vi "PH_ImageOperator.Fit Gauss.vi"(0 "No Offset?":bool, 1 "Diam":dbl, 2 "Trace":cluster{"Index":sgl[], "Trace":sgl[]}, 3 "calibrated?":bool, 4 "Order":i32, 5 "error in (no error)":errorcluster) -> (16 "Output":cluster{"Index":sgl[], "Best Fit":dbl[]}, 17 "mse":dbl format="%.2e", 18 "Best Fit Coefficients":dbl[](array[numeric]) format="%.2f", 19 "error out":errorcluster)   [LabVIEW 2014, in "PH_ImageOperator.lvlib"]
doc: "This VI fits a GAUSS function symmetrical to y-axis to the data connected to \"Trace\": a*exp(-(x/b))^2n + c\n\nwhere n is the \"Order\". To help the procedure, the \"Diameter\" (b) should be connected, while a first guess for a and c are extracted from the trace (maximum value and first value). The number of iterations is fixed to 20. The best (last) coefficients are given out as an array in the oder a, b, and c, as well as the medium square error (\"mse\")."
uses:
  PH_ImageOperator.lvlib
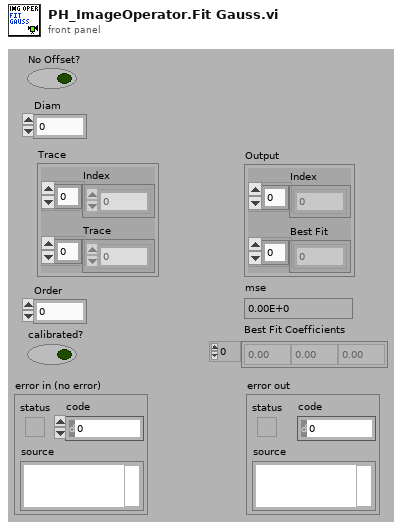
[diagram p1: front panel]
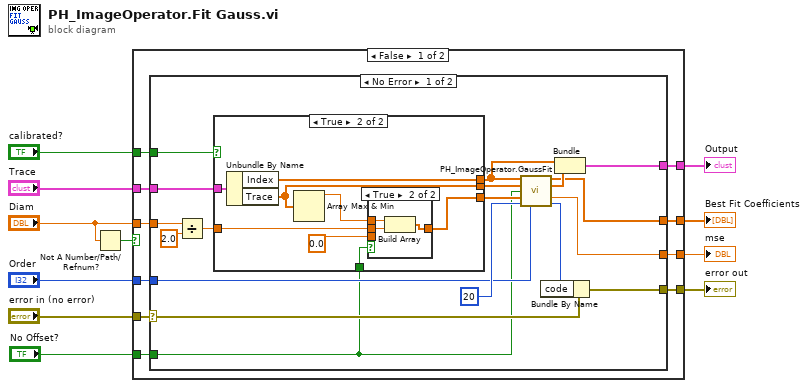
[diagram p0: block diagram]
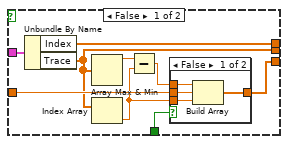
[diagram p2: hidden frame]
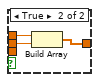
[diagram p3: hidden frame]
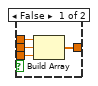
[diagram p4: hidden frame]
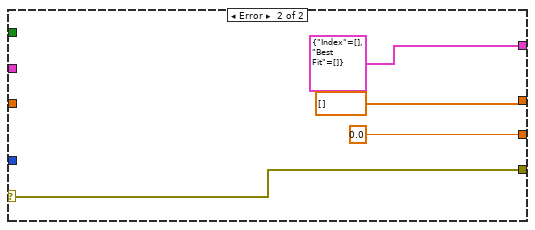
[diagram p5: hidden frame]
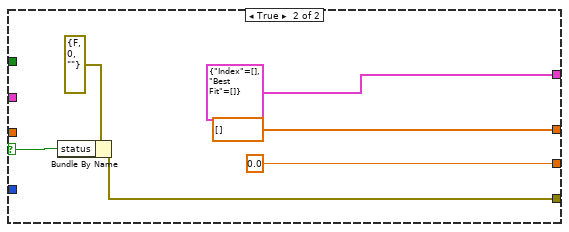
[diagram p6: hidden frame]
diagram:
  n1 = Not A Number/Path/Refnum?(number/path/refnum="Diam") -> (NaN/Path/Refnum?=w3:bool)
  n2 = case shown="False" w3 {
    selector: w3 -> [_ w78]
    tunnel: [w21 cluster{"Index":sgl[], "Best Fit":dbl[]} {"Index"=[], "Best Fit"=[]}] -> w11
    tunnel: "Trace" -> [w20 _]
    tunnel: "Order" -> [w19 _]
    tunnel: [w18 0.0 ("mse")] -> w8
    tunnel: [w17 dbl[] [] ("Best Fit Coefficients")] -> w7
    tunnel: "error in (no error)" -> [w16 _]
    tunnel: [w15 w79] -> w5
    tunnel: "Diam" -> [w14 _]
    tunnel: "calibrated?" -> [w13 _]
    tunnel: "No Offset?" -> [w12 _]
    frame False {
      n3 = case shown="No Error" w16 {
        selector: w16 -> [w28 w72]
        tunnel: w14 -> [w38 _]
        tunnel: [w34 cluster{"Index":sgl[], "Best Fit":dbl[]} {"Index"=[], "Best Fit"=[]}] -> w21
        tunnel: w20 -> [w31 _]
        tunnel: w19 -> [w23 _]
        tunnel: [w30 0.0 ("mse")] -> w18
        tunnel: [w29 dbl[] [] ("Best Fit Coefficients")] -> w17
        tunnel: [w27 w72] -> w15
        tunnel: w13 -> [w25 _]
        tunnel: w12 -> [w22 _]
        frame No Error {
          n4 = Divide(x=w38, y=2.0) -> (x/y=w37:dbl)
          n5 = case shown="True" w25 {
            tunnel: w37 -> [w48 w63]
            tunnel: [w47 w61] -> w36
            tunnel: [w46 w60] -> w35
            tunnel: [w45 w59] -> w33
            tunnel: w31 -> [w44 w58]
            tunnel: w22 -> [w40 w56]
            frame False {
              n6 = Unbundle By Name(w44) -> ("Index"=w45:sgl[], "Trace"=w47:sgl[])
              n7 = Array Max & Min(array=w47) -> (max value=w42:sgl)  [unwired: 3 out]
              n8 = Index Array(array=w47) -> (element=w43:sgl)  [unwired: 1 in]
              n9 = Subtract(x=w42, y=w43) -> (x-y=w41:sgl)
              n10 = case shown="False" w40 {
                tunnel: w48 -> [w52 w55]
                tunnel: [w51 w54] -> w46
                tunnel: w43 -> [w50 _]
                tunnel: w41 -> [w49 w53]
                frame False {
                  n11 = Build Array(w49, w52, w50) -> (w51:dbl[])
                }
                frame True {
                  n12 = Build Array(w53, w55) -> (w54:dbl[])
                }
              }
            }
            frame True {
              n13 = Unbundle By Name(w58) -> ("Index"=w59:sgl[], "Trace"=w61:sgl[])
              n14 = Array Max & Min(array=w61) -> (max value=w62:sgl)  [unwired: 3 out]
              n15 = case shown="True" w56 {
                tunnel: w63 -> [w67 w70]
                tunnel: w62 -> [w66 w69]
                tunnel: [w65 w68] -> w60
                tunnel: 0.0 ("element") -> [w64 _]
                frame False {
                  n16 = Build Array(w66, w67, w64) -> (w65:dbl[])
                }
                frame True {
                  n17 = Build Array(w69, w70) -> (w68:dbl[])
                }
              }
            }
          }
          n18 = call "PH_ImageOperator.GaussFit.vi"("Index"=w33, "Trace"=w36, "No Offset?"=w22, "Initial Guess Coefficients"=w35, "max iteration"=20, "Order of GAUSSian function"=w23) -> ("Best Fit Coefficients"=w29:dbl[], "Best Fit"=w32:dbl[], "mse"=w30:dbl, "error"=w26:i32)  [unwired: 5 in, 1 out]
          n19 = Bundle By Name(cluster=w28, "code"=w26) -> (w27:errorcluster)
          n20 = Bundle("Index"=w33, "Best Fit"=w32) -> (w34:cluster{"Index":sgl[], "Best Fit":dbl[]})  [unwired: 1 in]
        }
        frame Error {
        }
      }
    }
    frame True {
      n21 = Bundle By Name(cluster=errorcluster {"status"=FALSE, "code"=0, "source"=""} ("error IO"), "status"=w78) -> (w79:errorcluster)
    }
  }
  "Output" <- w11
  "mse" <- w8
  "Best Fit Coefficients" <- w7
  "error out" <- w5
